vi "Data Table Handler.vi"(0 "TableRef":refnum<vi>, 7 "DesiredRow":i32, 11 "TableRows":i32) -> (4 "RowIndex":i32)   [LabVIEW 2019]
uses:
  <vilib>/Utility/miscctls.llb/LVRowAndColumnTypeDef.ctl
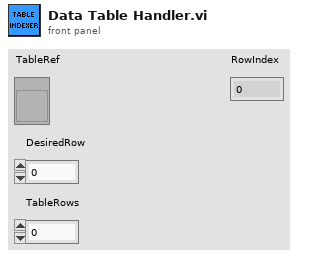
[diagram p1: front panel]
types:
  T1 = typedef "LVRowAndColumnUnsignedTypeDef.ctl" = cluster{"Row":u32, "Column":u32}
  T2 = typedef "LVRowAndColumnTypeDef.ctl" = cluster{"Row":i32, "Column":i32}
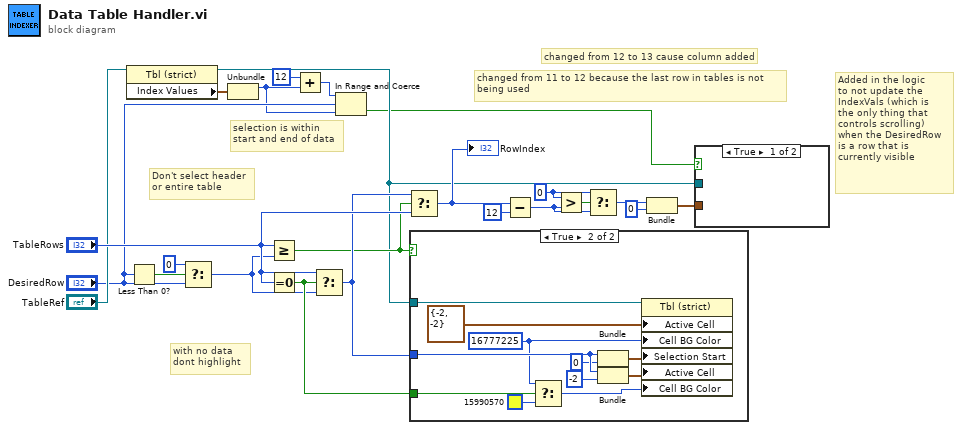
[diagram p0: block diagram]
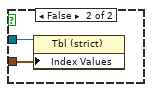
[diagram p2: hidden frame]
diagram:
  w21 = 0 ("y")
  # "changed from 12 to 13 cause column added"
  # "Added in the logic\nto not update the\nIndexVals (which is\nthe only thing that\ncontrols scrolling)\nwhen the DesiredRow\nis a row that is\ncurrently visible"
  # "changed from 11 to 12 because the last row in tables is not\nbeing used"
  # "with no data\ndont highlight"
  # "selection is within\nstart and end of data"
  # "Don't select header\nor entire table"
  n1 = property on="Property Node" class="Tbl (strict)"(reference="TableRef") -> (reference out=w7:refnum<vi>, "Index Values"=w6:T1)  [unwired: 1 in, 1 out]
  n2 = Less Than 0?(x="DesiredRow") -> (x < 0?=w11:bool)
  n3 = Select(t=0, s=w11, f="DesiredRow") -> (s? t:f=w9:i32)
  n4 = Unbundle(w6) -> ("Row"=w3:u32)  [unwired: 1 out]
  n5 = Greater Or Equal?(x="TableRows", y=w9) -> (x >= y?=w13:bool)
  n6 = Equal To 0?(x="TableRows") -> (x = 0?=w12:bool)
  n7 = Add(x=12 ("y"), y=w3) -> (x+y=w2:u32)
  n8 = Select(t="TableRows", s=w12, f=w9) -> (s? t:f=w14:i32)
  n9 = In Range and Coerce(upper limit=w2, x="DesiredRow", lower limit=w3) -> (In Range?=w1:bool)  [unwired: 1 out]
  n10 = Select(t=w14, s=w13, f="TableRows") -> (s? t:f=w19:i32)
  "RowIndex" <- w19
  n11 = case shown="True" w13 {
    tunnel: w14 -> [_ w31]
    tunnel: w7 -> [_ w28]
    tunnel: w12 -> [_ w27]
    frame False {
    }
    frame True {
      w26 = u32 16777225 ("Active Cell:Cell Background Color")
      n12 = Select(t=w26, s=w27, f=u32 15990570) -> (s? t:f=w24:u32)
      n13 = Bundle("DesiredRow"=w31, "y"=0) -> (w34:cluster{"DesiredRow":i32, "y":i32})  [unwired: 1 in]
      n14 = Bundle("DesiredRow"=w31, -2) -> (w33:cluster{"DesiredRow":i32, i32})  [unwired: 1 in]
      n15 = property on="Property Node" class="Tbl (strict)"(reference=w28, "Active Cell"=T2 {"Row"=-2, "Column"=-2} ("Active Cell:Active Cell"), "Cell BG Color"=w26, "Selection Start"=w34, "Active Cell"=w33, "Cell BG Color"=w24) -> ()  [unwired: 1 in, 2 out]
    }
  }
  n16 = Subtract(x=w19, y=12) -> (x-y=w22:i32)
  n17 = Greater?(x=w21, y=w22) -> (0:w23:bool)
  n18 = Select(t=w21, s=w23, f=w22) -> (s? t:f=w17:i32)
  n19 = Bundle("y"=w17, "y"=0) -> (w16:cluster{"y":i32, "y":i32})  [unwired: 1 in]
  n20 = case shown="True" w1 {
    tunnel: w16 -> [_ w36]
    tunnel: w7 -> [_ w35]
    frame True {
    }
    frame False {
      n21 = property on="Property Node" class="Tbl (strict)"(reference=w35, "Index Values"=w36) -> ()  [unwired: 1 in, 2 out]
    }
  }
